vi "bigcryo_H-full_ver2p1.vi"() -> ()   [LabVIEW 2019]
uses:
  Components/B_Globals.vi
  <vilib>/Analysis/NI_AALPro.lvlib
panel:
  in  "Heater On":bool
  in  "Pause Off":bool
  out "Set Field [T]":dbl=0.05
  out "Set Rate [T]":dbl=0.012520565999999999
  out "Exec Time [ms]":u32=400
  out "Stable":bool
  out "Act. Rate [T/min]":dbl=-0.0
  out "Read Buffer":string="15:13:43 OUTPUT: 0.00000 TESLA AT 0.0 VOLTS\r\n"
  in  "stop":bool
  out "Its":i32=50
  out "Running Sequence":bool
  in  "Set Field":dbl
  in  "Rate":dbl=0.05
  in  "Go To":bool
  out "Field [T]":dbl
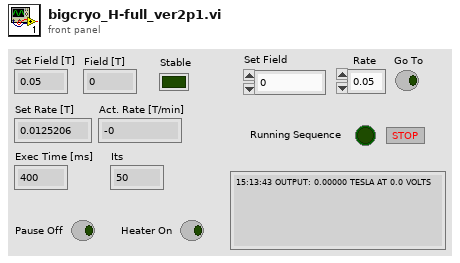
[diagram p1: front panel]
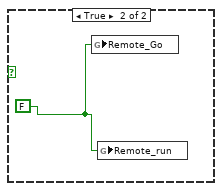
[diagram p2: hidden frame]
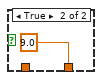
[diagram p5: hidden frame]
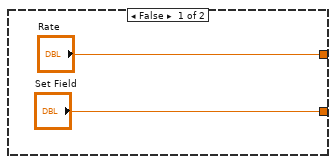
[diagram p7: hidden frame]
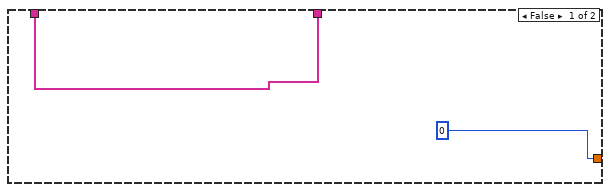
[diagram p9: hidden frame]
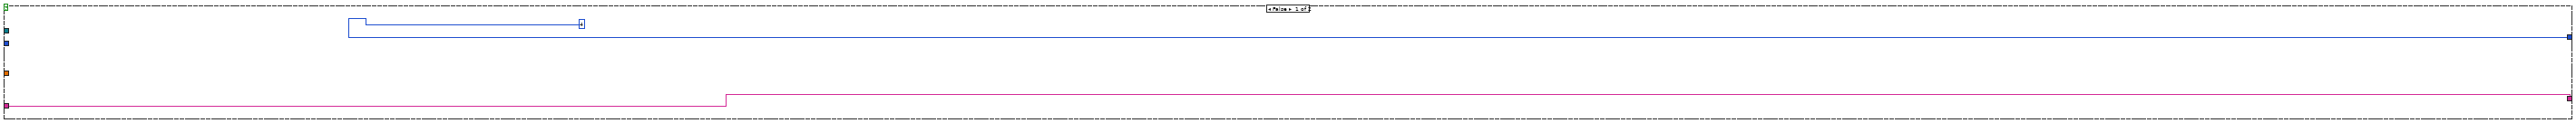
[diagram p12: hidden frame]
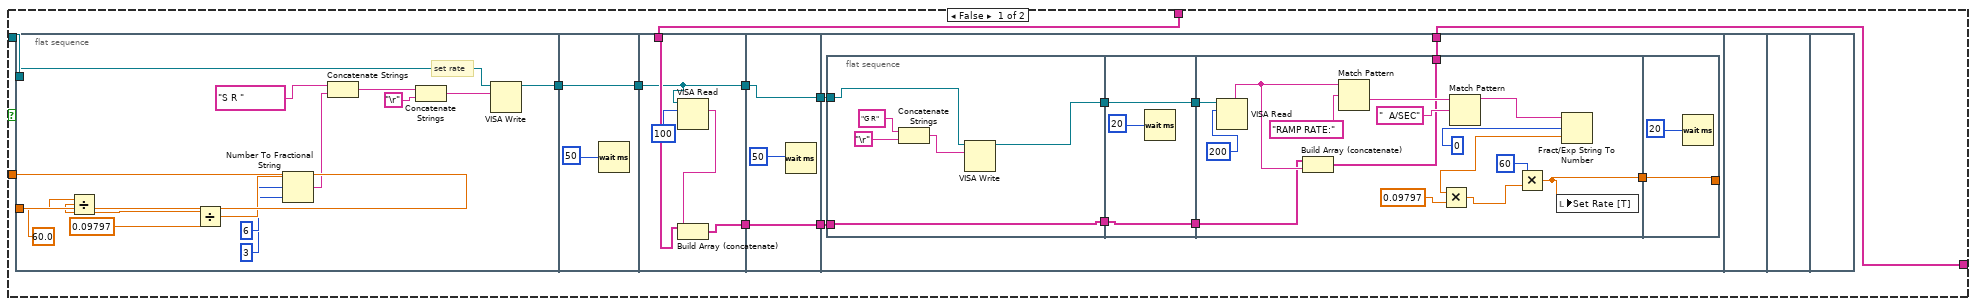
[diagram p13: hidden frame]
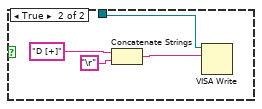
[diagram p17: hidden frame]
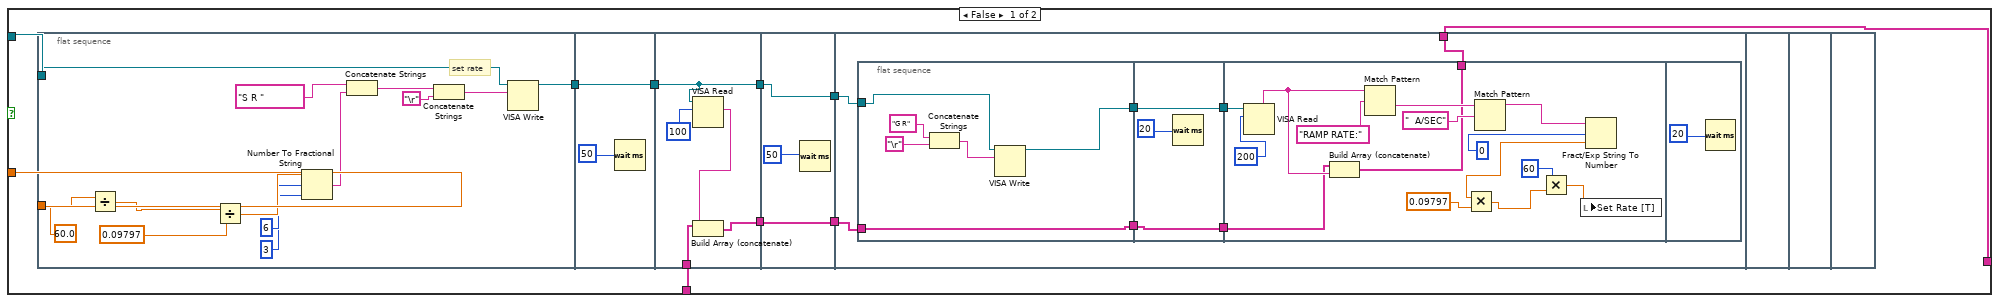
[diagram p18: hidden frame]
diagram:
  n1 = Tick Count (ms)() -> (millisecond timer value=w1:u32)
  n2 = VISA Clear(VISA resource name=refnum<visa-resource-name> "COM6" ("Lakeshore Address")) -> (VISA resource name out=w3:refnum<visa-resource-name>)  [unwired: 1 in, 1 out]
  n3 = while {
    shift-right: [w103] -> _
    shift-left: _ -> [w104]
    shift-right: [w100] -> _
    shift-left: _ -> [w101]
    tunnel: w3 -> [w105]
    shift-right: [w96] -> _
    shift-left: 0 -> [w50]
    shift-right: [w83] -> _
    shift-left: w1 -> [w82]
    shift-right: [w23] -> _
    shift-left: _ -> [w34]
    i -> [w93]
    stop <- FALSE stop-if-true
    n4 = flat-sequence {
      tunnel: w50 -> [w114]
      tunnel: w101 -> [w108]
      tunnel: w104 -> [w110]
      tunnel: w105 -> [w115]
      tunnel: [w115] -> w49
      tunnel: [w111] -> w48
      tunnel: [w107] -> w47
      tunnel: [w114] -> w46
      tunnel: [w106] -> w35
      tunnel: w34 -> [w106]
      tunnel: [w123] -> w87
      tunnel: [w122] -> w86
      tunnel: [w121] -> w85
      tunnel: [w120] -> w84
      tunnel: [w118] -> w83
      tunnel: w82 -> [w117]
      tunnel: w49 -> [w123]
      tunnel: w48 -> [w122]
      tunnel: w47 -> [w121]
      tunnel: w46 -> [w120]
      tunnel: w35 -> [w116]
      tunnel: [w116] -> w31
      tunnel: [w130] -> w45
      tunnel: [w129] -> w43
      tunnel: [w128] -> w41
      tunnel: [w127] -> w39
      tunnel: [w125] -> w37
      tunnel: w87 -> [w130]
      tunnel: w86 -> [w129]
      tunnel: w85 -> [w128]
      tunnel: w84 -> [w127]
      tunnel: [w124] -> w32
      tunnel: w31 -> [w124]
      tunnel: w45 -> [w134]
      tunnel: [w133] -> w44
      tunnel: w43 -> [w138]
      tunnel: [w138] -> w42
      tunnel: w41 -> [w137]
      tunnel: [w137] -> w40
      tunnel: w39 -> [w136]
      tunnel: [w136] -> w38
      tunnel: w37 -> [w135]
      tunnel: [w135] -> w36
      tunnel: [w132] -> w33
      tunnel: w32 -> [w132]
      tunnel: w44 -> [w141]
      tunnel: [w140] -> w92
      tunnel: w42 -> [w148]
      tunnel: [w148] -> w91
      tunnel: w40 -> [w147]
      tunnel: [w147] -> w90
      tunnel: w38 -> [w146]
      tunnel: [w146] -> w89
      tunnel: w36 -> [w145]
      tunnel: [w145] -> w88
      tunnel: w33 -> [w144]
      tunnel: [w144] -> w29
      tunnel: [w198] -> w81
      tunnel: [w197] -> w80
      tunnel: [w195] -> w79
      tunnel: [w196] -> w78
      tunnel: [w191] -> w77
      tunnel: w92 -> [w191]
      tunnel: w91 -> [w198]
      tunnel: w90 -> [w197]
      tunnel: w89 -> [w196]
      tunnel: w88 -> [w195]
      tunnel: [w190] -> w51
      tunnel: [w189] -> w30
      tunnel: w29 -> [w189]
      tunnel: w81 -> [w206]
      tunnel: [w206] -> w76
      tunnel: w80 -> [w205]
      tunnel: [w205] -> w75
      tunnel: w79 -> [w204]
      tunnel: [w204] -> w74
      tunnel: w78 -> [w203]
      tunnel: [w203] -> w73
      tunnel: w77 -> [w202]
      tunnel: [w202] -> w72
      tunnel: [w200] -> w52
      tunnel: w51 -> [w200]
      tunnel: w30 -> [w199]
      tunnel: [w199] -> w27
      tunnel: [w210] -> w71
      tunnel: w76 -> [w221]
      tunnel: [w221] -> w70
      tunnel: w75 -> [w220]
      tunnel: [w220] -> w69
      tunnel: w74 -> [w219]
      tunnel: [w219] -> w68
      tunnel: w73 -> [w218]
      tunnel: [w218] -> w67
      tunnel: w72 -> [w217]
      tunnel: [w217] -> w66
      tunnel: [w209] -> w65
      tunnel: w52 -> [w208]
      tunnel: [w207] -> w28
      tunnel: w27 -> [w207]
      tunnel: [w230] -> w64
      tunnel: [w225] -> w62
      tunnel: [w229] -> w60
      tunnel: [w228] -> w58
      tunnel: [w227] -> w56
      tunnel: [w226] -> w54
      tunnel: w71 -> [w225]
      tunnel: w70 -> [w226]
      tunnel: w69 -> [w228]
      tunnel: w68 -> [w227]
      tunnel: w67 -> [w230]
      tunnel: w66 -> [w229]
      tunnel: w65 -> [w224]
      tunnel: w28 -> [w222]
      tunnel: [w223] -> w25
      tunnel: w64 -> [w238]
      tunnel: [w238] -> w63
      tunnel: w62 -> [w237]
      tunnel: [w237] -> w61
      tunnel: w60 -> [w236]
      tunnel: [w236] -> w59
      tunnel: w58 -> [w235]
      tunnel: [w235] -> w57
      tunnel: w56 -> [w234]
      tunnel: [w234] -> w55
      tunnel: w54 -> [w233]
      tunnel: [w233] -> w53
      tunnel: [w231] -> w26
      tunnel: w25 -> [w231]
      tunnel: [w265] -> w99
      tunnel: [w263] -> w98
      tunnel: [w273] -> w97
      tunnel: w63 -> [w273]
      tunnel: [w268] -> w95
      tunnel: w61 -> [w268]
      tunnel: [w272] -> w94
      tunnel: w59 -> [w272]
      tunnel: w57 -> [w271]
      tunnel: w55 -> [w270]
      tunnel: w53 -> [w269]
      tunnel: w26 -> [w256]
      tunnel: [w256] -> w24
      tunnel: w99 -> [w292]
      tunnel: w98 -> [w291]
      tunnel: w97 -> [w287]
      tunnel: [w292] -> w22
      tunnel: [w291] -> w20
      tunnel: [w286] -> w18
      tunnel: [w285] -> w16
      tunnel: w95 -> [w285]
      tunnel: w94 -> [w284]
      tunnel: [w284] -> w14
      tunnel: [w274] -> w12
      tunnel: [w278] -> w10
      tunnel: [w282] -> w8
      tunnel: w24 -> [w282]
      tunnel: w22 -> [w320]
      tunnel: [w320] -> w21
      tunnel: w20 -> [w319]
      tunnel: [w319] -> w19
      tunnel: w18 -> [w306]
      tunnel: [w306] -> w17
      tunnel: w16 -> [w318]
      tunnel: [w318] -> w15
      tunnel: w14 -> [w315]
      tunnel: [w315] -> w13
      tunnel: w12 -> [w317]
      tunnel: [w317] -> w11
      tunnel: w10 -> [w316]
      tunnel: [w316] -> w9
      tunnel: w8 -> [w314]
      tunnel: [w313] -> w7
      tunnel: [w311] -> w6
      tunnel: [w309] -> w5
      tunnel: [w364] -> w100
      tunnel: [w365] -> w103
      tunnel: w21 -> [w365]
      tunnel: w19 -> [w364]
      tunnel: w17 -> [w358]
      tunnel: [w363] -> w96
      tunnel: w15 -> [w362]
      tunnel: w13 -> [w361]
      tunnel: w11 -> [w360]
      tunnel: w9 -> [w359]
      tunnel: [w357] -> w23
      tunnel: w7 -> [w356]
      tunnel: w6 -> [w355]
      tunnel: w5 -> [w354]
      frame #0 {
        n5 = Array Size(array=w110) -> (size(s)=w113:i32)
        n6 = Subtract(x=w113, y=1000) -> (x-y=w109:i32)
        n7 = Array Subset(array=w110, index=w109) -> (w111:dbl[])  [unwired: 1 in]
        n8 = Array Subset(array=w108, index=w109) -> (w107:dbl[])  [unwired: 1 in]
      }
      frame #1 {
        n9 = Tick Count (ms)() -> (millisecond timer value=w118:u32)
        n10 = Subtract(x=w118, y=w117) -> (x-y=→"Exec Time [ms]":u32)
      }
      frame #2 {
        n11 = case shown="False" "stop" {
          frame False {
          }
          frame True {
            w131 = FALSE
            n12 = global write "B_Globals.vi" "Remote_Go"(w131) -> ()
            n13 = global write "B_Globals.vi" "Remote_run"(w131) -> ()
          }
        }
        n14 = call <vilib>:"High Resolution Relative Seconds.vi"() -> ("relative seconds"=w125:dbl)
      }
      frame #3 {
        n15 = VISA Clear(VISA resource name=w134) -> (VISA resource name out=w133:refnum<visa-resource-name>)  [unwired: 1 in, 1 out]
      }
      frame #4 {
        n16 = case shown="True" "Pause Off" {
          tunnel: w141 -> [w169 w170]
          tunnel: [w169 w173] -> w139
          frame False {
          }
          frame True {
            n17 = flat-sequence {
              tunnel: [w176] -> w172
              tunnel: w170 -> [w175]
              tunnel: w172 -> [w180]
              tunnel: [w180] -> w171
              tunnel: [w185] -> w174
              tunnel: w171 -> [w184]
              tunnel: [w186] -> _
              tunnel: w174 -> [w186]
              tunnel: [w186] -> w173
              frame #0 {
                n18 = Concatenate Strings("P  [0]" ("Command"), "\r") -> (w178:string)
                n19 = VISA Write(VISA resource name=w175, write buffer=w178) -> (VISA resource name out=w176:refnum<visa-resource-name>)  [unwired: 1 in, 2 out]
              }
              frame #1 {
                n20 = Wait (ms)(milliseconds to wait=u32 50 ("Pre Delay")) -> ()  [unwired: 1 out]
              }
              frame #2 {
                n21 = VISA Read(VISA resource name=w184, byte count=u32 200) -> (VISA resource name out=w185:refnum<visa-resource-name>, read buffer=w182:string)  [unwired: 1 in, 2 out]
                n22 = local write "Read Buffer"(w182) -> ()
              }
              frame #3 {
                n23 = Wait (ms)(milliseconds to wait=u32 50 ("Pre Delay")) -> ()  [unwired: 1 out]
                n24 = local write "Pause Off"(FALSE) -> ()
              }
            }
          }
        }
        n25 = case shown="True" "Heater On" {
          tunnel: [w149 w150] -> w140
          tunnel: w139 -> [w149 w151]
          frame False {
          }
          frame True {
            n26 = flat-sequence {
              tunnel: [w156] -> w154
              tunnel: w151 -> [w155]
              tunnel: w154 -> [w160]
              tunnel: [w160] -> w153
              tunnel: [w165] -> w152
              tunnel: w153 -> [w164]
              tunnel: [w166] -> w150
              tunnel: w152 -> [w166]
              tunnel: [w166] -> _
              frame #0 {
                n27 = Concatenate Strings("H  [1]" ("Command"), "\r") -> (w158:string)
                n28 = VISA Write(VISA resource name=w155, write buffer=w158) -> (VISA resource name out=w156:refnum<visa-resource-name>)  [unwired: 1 in, 2 out]
              }
              frame #1 {
                n29 = Wait (ms)(milliseconds to wait=u32 50 ("Pre Delay")) -> ()  [unwired: 1 out]
              }
              frame #2 {
                n30 = VISA Read(VISA resource name=w164, byte count=u32 200) -> (VISA resource name out=w165:refnum<visa-resource-name>, read buffer=w162:string)  [unwired: 1 in, 2 out]
                n31 = local write "Read Buffer"(w162) -> ()
              }
              frame #3 {
                n32 = Wait (ms)(milliseconds to wait=u32 50 ("Pre Delay")) -> ()  [unwired: 1 out]
                n33 = local write "Heater On"(FALSE) -> ()
              }
            }
          }
        }
      }
      frame #5 {
        n34 = Concatenate Strings("G O" ("Command"), "\r") -> (w193:string)
        n35 = VISA Write(VISA resource name=w191, write buffer=w193) -> (VISA resource name out=w190:refnum<visa-resource-name>)  [unwired: 1 in, 2 out]
      }
      frame #6 {
        n36 = Wait (ms)(milliseconds to wait=u32 50 ("Pre Delay")) -> ()  [unwired: 1 out]
      }
      frame #7 {
        n37 = VISA Read(VISA resource name=w208, byte count=u32 200) -> (read buffer=w209:string)  [unwired: 1 in, 3 out]
        n38 = Match Pattern(string=w209, regular expression="OUTPUT:") -> (after substring=w212:string)  [unwired: 1 in, 3 out]
        n39 = Match Pattern(string=w212, regular expression=" TESLA") -> (before substring=w211:string)  [unwired: 1 in, 3 out]
        n40 = Fract/Exp String To Number(string=w211, offset=0) -> (number=w210:dbl)  [unwired: 2 in, 1 out]
      }
      frame #8 {
        n41 = global write "B_Globals.vi" "B [T]"(w225) -> ()
        n42 = Build Array (concatenate)(w222, w224) -> (w223:string[])
        "Field [T]" <- w225
        "Read Buffer" <- w224
      }
      frame #9 {
        n43 = Wait (ms)(milliseconds to wait=u32 50 ("Pre Delay")) -> ()  [unwired: 1 out]
      }
      frame #10 {
        n44 = Build Array (concatenate)(w269, w268) -> (w265:dbl[])
        n45 = Build Array (concatenate)(w271, w270) -> (w263:dbl[])
        n46 = Array Size(array=w265) -> (size(s)=w266:i32)
        n47 = Subtract(x=w266, y=50) -> (x-y=w264:i32)
        n48 = Array Subset(array=w263, index=w264) -> (w261:dbl[])  [unwired: 1 in]
        n49 = Array Subset(array=w265, index=w264) -> (w262:dbl[])  [unwired: 1 in]
        n50 = local read "Set Field [T]"() -> (w250:dbl)
        n51 = call <vilib>:"Linear Fit.vi"("Y"=w262, "X"=w261) -> ("slope"=w258:dbl)  [unwired: 9 in, 4 out]
        n52 = local read "Field [T]"() -> (w248:dbl)
        n53 = Multiply(x=w258, y=60) -> (x*y=w257:dbl)
        "Act. Rate [T/min]" <- w257
        n54 = Absolute Value(x=w250) -> (abs(x)=w249:dbl)
        n55 = Absolute Value(x=w248) -> (abs(x)=w240:dbl)
        n56 = Add(x=1, y=w240) -> (x+y=w239:dbl)
        n57 = Multiply(x=0.008, y=w239) -> (x*y=w246:dbl)
        n58 = Subtract(x=w249, y=w240) -> (x-y=w255:dbl)
        n59 = Absolute Value(x=w257) -> (abs(x)=w259:dbl)
        n60 = Less?(x=w259, y=w246) -> (x < y?=w252:bool)
        n61 = Add(x=1, y=w240) -> (x+y=w242:dbl)
        n62 = Absolute Value(x=w255) -> (abs(x)=w254:dbl)
        n63 = Multiply(x=w242, y=0.008) -> (x*y=w244:dbl)
        n64 = Less?(x=w254, y=w244) -> (x < y?=w251:bool)
        n65 = And(x=w252, y=w251) -> (x .and. y?=w253:bool)
        "Stable" <- w253
        n66 = global write "B_Globals.vi" "Rem_stable_B"(w253) -> ()
      }
      frame #11 {
        n67 = global read "B_Globals.vi" "Remote_Go"() -> (w290:bool)
        n68 = global read "B_Globals.vi" "Remote_run"() -> (w283:bool)
        "Running Sequence" <- w283
        n69 = Or(x=w290, y="Go To") -> (x .or. y?=w288:bool)
        n70 = case shown="True" w288 {
          tunnel: w287 -> [w301 w303]
          tunnel: [w301 w302] -> w286
          frame False {
          }
          frame True {
            n71 = flat-sequence {
              tunnel: w303 -> [_]
              tunnel: [1] -> w302
              frame #0 {
              }
              frame #1 {
                w305 = FALSE
                n72 = local write "Go To"(w305) -> ()
                n73 = global write "B_Globals.vi" "Remote_Go"(w305) -> ()
              }
            }
          }
        }
        n74 = case shown="True" w283 {
          tunnel: ["Set Field" w299] -> w275
          tunnel: ["Rate" w300] -> w279
          frame False {
          }
          frame True {
            n75 = global read "B_Globals.vi" "Remote_Rate"() -> (w300:dbl)
            n76 = global read "B_Globals.vi" "Remote_set"() -> (w299:dbl)
            n77 = local write "Rate"(w300) -> ()
            n78 = local write "Set Field"(w299) -> ()
          }
        }
        n79 = Greater?(x=w279, y=0.5) -> (0:w280:bool)
        n80 = Greater?(x=w275, y=9.0) -> (0:w276:bool)
        n81 = case shown="False" w276 {
          tunnel: [w293 9.0] -> w274
          tunnel: w275 -> [w293 _]
          frame False {
          }
          frame True {
          }
        }
        n82 = case shown="True" w280 {
          tunnel: [w295 0.5] -> w278
          tunnel: w279 -> [w295 _]
          frame False {
          }
          frame True {
          }
        }
      }
      frame #12 {
        n83 = Not Equal?(x=0, y=w306) -> (x != y?=w309:bool)
        n84 = Not Equal?(x=w306, y=2) -> (x != y?=w310:bool)
        n85 = And(x=w309, y=w310) -> (x .and. y?=w308:bool)
        n86 = case shown="True" w308 {
          tunnel: w315 -> [_ w327]
          tunnel: w314 -> [w322 w326]
          tunnel: [w322 w325] -> w313
          tunnel: [0 w323] -> w311
          frame False {
          }
          frame True {
            n87 = flat-sequence {
              tunnel: w327 -> [w331]
              tunnel: [w330] -> w329
              tunnel: w329 -> [w335]
              tunnel: [w335] -> w328
              tunnel: w328 -> [w348]
              tunnel: w326 -> [w345]
              tunnel: [w344] -> w325
              tunnel: [w337] -> w324
              tunnel: [w352] -> w323
              tunnel: w324 -> [w352]
              frame #0 {
                n88 = Concatenate Strings("G R" ("Command"), "\r") -> (w333:string)
                n89 = VISA Write(VISA resource name=w331, write buffer=w333) -> (VISA resource name out=w330:refnum<visa-resource-name>)  [unwired: 1 in, 2 out]
              }
              frame #1 {
                n90 = Wait (ms)(milliseconds to wait=20) -> ()  [unwired: 1 out]
              }
              frame #2 {
                n91 = VISA Read(VISA resource name=w348, byte count=u32 200) -> (read buffer=w346:string)  [unwired: 1 in, 3 out]
                n92 = Build Array (concatenate)(w345, w346) -> (w344:string[])
                n93 = Match Pattern(string=w346, regular expression="RAMP RATE:") -> (after substring=w349:string)  [unwired: 1 in, 3 out]
                n94 = Match Pattern(string=w349, regular expression="  A/SEC") -> (before substring=w342:string)  [unwired: 1 in, 3 out]
                n95 = Fract/Exp String To Number(string=w342, offset=0) -> (number=w340:dbl)  [unwired: 2 in, 1 out]
                n96 = Multiply(x=w340, y=0.09797) -> (x*y=w338:dbl)
                n97 = Multiply(x=60, y=w338) -> (x*y=w337:dbl)
                "Set Rate [T]" <- w337
              }
              frame #3 {
                n98 = Wait (ms)(milliseconds to wait=20) -> ()  [unwired: 1 out]
              }
            }
          }
        }
      }
      frame #13 {
        # "Bnow"
        # "Barray"
        n99 = case shown="4" w358 {
          tunnel: w362 -> [_ w384 w591 _ _]
          tunnel: w358 -> [w368 w377 w588 _ _]
          tunnel: [w368 w376 w587 4 w646] -> w363
          tunnel: w359 -> [_ w369 _ _ w648]
          tunnel: w361 -> [_ w373 _ w600 w644]
          tunnel: w360 -> [_ w374 _ _ w645]
          tunnel: w356 -> [w366 w372 w586 w598 w629]
          tunnel: [w366 w371 w586 w598 w623] -> w357
          tunnel: w355 -> [_ w370 _ _ _]
          tunnel: w354 -> [_ _ _ _ _]
          frame 0, Default {
            n100 = Wait (ms)(milliseconds to wait=0) -> ()  [unwired: 1 out]
          }
          frame 1 {
            # "If True need to reverse polarity"
            n101 = Less Than 0?(x=w374) -> (x < 0?=w375:bool)
            n102 = Number To Fractional String(number=w384) -> (F-format string=w387:string)  [unwired: 3 in]
            n103 = String Subset(string=w387, length (rest)=1 ("length (rest)")) -> (substring=w386:string)  [unwired: 1 in]
            n104 = Equal?(x=w386, y="-") -> (x = y?=w379:bool)
            n105 = Not Or(1:w375, 2:w379) -> (0:w383:bool)
            n106 = Not Or(1:w383, 2:w379) -> (0:w382:bool)
            n107 = Not Or(1:w375, 2:w383) -> (0:w381:bool)
            n108 = Not Or(1:w381, 2:w382) -> (0:w380:bool)
            n109 = Not(x=w380) -> (.not. x?=w378:bool)
            n110 = case shown="True" w378 {
              tunnel: w377 -> [_ _]
              tunnel: [4 2] -> w376
              tunnel: w369 -> [_ w438]
              tunnel: w373 -> [_ w436]
              tunnel: w372 -> [w389 w427]
              tunnel: [w389 w418] -> w371
              tunnel: w370 -> [_ w399]
              tunnel: w369 -> [_ w397]
              frame False {
              }
              frame True {
                n111 = flat-sequence {
                  tunnel: w436 -> [w442]
                  tunnel: [w442] -> w435
                  tunnel: [w443] -> w428
                  tunnel: w427 -> [w443]
                  tunnel: [w441] -> w400
                  tunnel: w399 -> [w441]
                  tunnel: [w446] -> w406
                  tunnel: w435 -> [w446]
                  tunnel: w428 -> [w445]
                  tunnel: [w445] -> w405
                  tunnel: w400 -> [w444]
                  tunnel: [w444] -> w398
                  tunnel: w406 -> [w454]
                  tunnel: [w454] -> w404
                  tunnel: w405 -> [w453]
                  tunnel: [w453] -> w402
                  tunnel: w398 -> [w452]
                  tunnel: w397 -> [w451]
                  tunnel: [w447] -> w396
                  tunnel: w404 -> [w457]
                  tunnel: [w457] -> w403
                  tunnel: w402 -> [w456]
                  tunnel: [w456] -> w401
                  tunnel: w396 -> [w455]
                  tunnel: [w455] -> w395
                  tunnel: [w462] -> w439
                  tunnel: w403 -> [w461]
                  tunnel: [w460] -> w425
                  tunnel: w401 -> [w460]
                  tunnel: [w459] -> w407
                  tunnel: w395 -> [w458]
                  tunnel: [w458] -> w394
                  tunnel: [w473] -> w434
                  tunnel: w439 -> [w473]
                  tunnel: [w472] -> w426
                  tunnel: w425 -> [w472]
                  tunnel: [w471] -> w408
                  tunnel: w407 -> [w471]
                  tunnel: w394 -> [w470]
                  tunnel: [w470] -> w393
                  tunnel: w434 -> [w485]
                  tunnel: [w485] -> w433
                  tunnel: w426 -> [w484]
                  tunnel: [w483] -> w423
                  tunnel: [w475] -> w409
                  tunnel: w408 -> [_]
                  tunnel: w393 -> [w482]
                  tunnel: [w482] -> w392
                  tunnel: w433 -> [w491]
                  tunnel: [w491] -> w432
                  tunnel: [w489] -> w424
                  tunnel: w423 -> [w489]
                  tunnel: [w488] -> w410
                  tunnel: w409 -> [w488]
                  tunnel: w392 -> [w487]
                  tunnel: [w487] -> w391
                  tunnel: w432 -> [w492]
                  tunnel: w438 -> [w497]
                  tunnel: [w492] -> w437
                  tunnel: w424 -> [w493]
                  tunnel: [w494] -> w421
                  tunnel: [w496] -> w411
                  tunnel: w410 -> [w496]
                  tunnel: w391 -> [w495]
                  tunnel: [w569] -> w431
                  tunnel: w437 -> [w569]
                  tunnel: [w568] -> w422
                  tunnel: w421 -> [w568]
                  tunnel: [w567] -> w412
                  tunnel: w411 -> [w567]
                  tunnel: w431 -> [w572]
                  tunnel: [w572] -> w430
                  tunnel: w422 -> [w570]
                  tunnel: [w570] -> w419
                  tunnel: [w571] -> w413
                  tunnel: w412 -> [w571]
                  tunnel: w430 -> [w575]
                  tunnel: [w575] -> w429
                  tunnel: [w574] -> w420
                  tunnel: w419 -> [w574]
                  tunnel: [w573] -> w414
                  tunnel: w413 -> [w573]
                  tunnel: w429 -> [w578]
                  tunnel: w420 -> [w577]
                  tunnel: [w577] -> w417
                  tunnel: [w576] -> w415
                  tunnel: w414 -> [w576]
                  tunnel: w417 -> [w583]
                  tunnel: [w583] -> w416
                  tunnel: w415 -> [w582]
                  tunnel: [w584] -> w418
                  tunnel: w416 -> [w584]
                  frame #0 {
                  }
                  frame #1 {
                  }
                  frame #2 {
                    n112 = Subtract(x=w452, y=w451) -> (x-y=w450:dbl)
                    n113 = Absolute Value(x=w450) -> (abs(x)=w449:dbl)
                    n114 = Less?(x=w449, y=0.01) -> (x < y?=w447:bool)
                  }
                  frame #3 {
                  }
                  frame #4 {
                    w459 = 0.0
                    # "set set field"
                    n115 = Number To Fractional String(number=w459, width (-)=i16 6, precision (6)=i16 3) -> (F-format string=w466:string)  [unwired: 1 in]
                    n116 = Concatenate Strings("S [%][MID] " ("string"), w466) -> (w463:string)
                    n117 = Concatenate Strings(w463, "\r") -> (w465:string)
                    n118 = VISA Write(VISA resource name=w461, write buffer=w465) -> (VISA resource name out=w462:refnum<visa-resource-name>)  [unwired: 1 in, 2 out]
                  }
                  frame #5 {
                    n119 = Wait (ms)(milliseconds to wait=50) -> ()  [unwired: 1 out]
                  }
                  frame #6 {
                    n120 = VISA Read(VISA resource name=w485, byte count=100) -> (read buffer=w476:string)  [unwired: 1 in, 3 out]
                    n121 = Match Pattern(string=w476, regular expression="SETTING:") -> (after substring=w480:string)  [unwired: 1 in, 3 out]
                    n122 = local write "Read Buffer"(w476) -> ()
                    n123 = Match Pattern(string=w480, regular expression=" TESLA") -> (before substring=w481:string)  [unwired: 1 in, 3 out]
                    n124 = Build Array (concatenate)(w484, w476) -> (w483:string[])
                    n125 = Fract/Exp String To Number(string=w481, offset=0) -> (number=w475:dbl)  [unwired: 2 in, 1 out]
                  }
                  frame #7 {
                    n126 = Wait (ms)(milliseconds to wait=50) -> ()  [unwired: 1 out]
                  }
                  frame #8 {
                    n127 = case shown="True" w495 {
                      tunnel: w492 -> [w507 _]
                      tunnel: w497 -> [w506 _]
                      tunnel: w493 -> [w502 w566]
                      tunnel: [w499 w566] -> w494
                      frame False {
                        n128 = flat-sequence {
                          tunnel: w507 -> [w510]
                          tunnel: w506 -> [w509]
                          tunnel: [w508] -> w505
                          tunnel: w505 -> [w523]
                          tunnel: [w523] -> w504
                          tunnel: w504 -> [w525]
                          tunnel: [w525] -> w503
                          tunnel: w502 -> [w526]
                          tunnel: [w524] -> w500
                          tunnel: w503 -> [w529]
                          tunnel: [w530] -> w501
                          tunnel: w500 -> [w530]
                          tunnel: [w529] -> w498
                          tunnel: w501 -> [w536]
                          tunnel: [w533] -> w499
                          tunnel: w498 -> [w532]
                          frame #0 {
                            # "set rate"
                            n129 = Divide(x=w509, y=60.0) -> (x/y=w515:dbl)
                            n130 = Divide(x=w515, y=0.09797) -> (x/y=w513:dbl)
                            n131 = Number To Fractional String(number=w513, width (-)=i16 6, precision (6)=i16 3) -> (F-format string=w518:string)  [unwired: 1 in]
                            n132 = Concatenate Strings("S R " ("string"), w518) -> (w517:string)
                            n133 = Concatenate Strings(w517, "\r") -> (w521:string)
                            n134 = VISA Write(VISA resource name=w510, write buffer=w521) -> (VISA resource name out=w508:refnum<visa-resource-name>)  [unwired: 1 in, 2 out]
                          }
                          frame #1 {
                            n135 = Wait (ms)(milliseconds to wait=50) -> ()  [unwired: 1 out]
                          }
                          frame #2 {
                            n136 = VISA Read(VISA resource name=w525, byte count=100) -> (read buffer=w527:string)  [unwired: 1 in, 3 out]
                            n137 = Build Array (concatenate)(w526, w527) -> (w524:string[])
                          }
                          frame #3 {
                            n138 = Wait (ms)(milliseconds to wait=50) -> ()  [unwired: 1 out]
                          }
                          frame #4 {
                            n139 = flat-sequence {
                              tunnel: [w542] -> w539
                              tunnel: w536 -> [w541]
                              tunnel: [w541] -> w534
                              tunnel: w532 -> [w540]
                              tunnel: w539 -> [w547]
                              tunnel: [w547] -> w538
                              tunnel: [w546] -> w535
                              tunnel: w534 -> [w546]
                              tunnel: w538 -> [w560]
                              tunnel: [w557] -> w533
                              tunnel: [w550] -> w537
                              tunnel: w535 -> [w549]
                              tunnel: [w564] -> _
                              tunnel: w537 -> [w564]
                              frame #0 {
                                n140 = Concatenate Strings("G R" ("Command"), "\r") -> (w544:string)
                                n141 = VISA Write(VISA resource name=w540, write buffer=w544) -> (VISA resource name out=w542:refnum<visa-resource-name>)  [unwired: 1 in, 2 out]
                              }
                              frame #1 {
                                n142 = Wait (ms)(milliseconds to wait=20) -> ()  [unwired: 1 out]
                              }
                              frame #2 {
                                n143 = VISA Read(VISA resource name=w560, byte count=u32 200) -> (read buffer=w558:string)  [unwired: 1 in, 3 out]
                                n144 = Build Array (concatenate)(w549, w558) -> (w557:string[])
                                n145 = Match Pattern(string=w558, regular expression="RAMP RATE:") -> (after substring=w561:string)  [unwired: 1 in, 3 out]
                                n146 = Match Pattern(string=w561, regular expression="  A/SEC") -> (before substring=w555:string)  [unwired: 1 in, 3 out]
                                n147 = Fract/Exp String To Number(string=w555, offset=0) -> (number=w553:dbl)  [unwired: 2 in, 1 out]
                                n148 = Multiply(x=w553, y=0.09797) -> (x*y=w551:dbl)
                                n149 = Multiply(x=60, y=w551) -> (x*y=w550:dbl)
                                n150 = local write "Set Rate [T]"(w550) -> ()
                              }
                              frame #3 {
                                n151 = Wait (ms)(milliseconds to wait=20) -> ()  [unwired: 1 out]
                              }
                            }
                          }
                          frame #5 {
                          }
                          frame #6 {
                          }
                          frame #7 {
                          }
                        }
                      }
                      frame True {
                      }
                    }
                  }
                  frame #9 {
                  }
                  frame #10 {
                  }
                  frame #11 {
                  }
                  frame #12 {
                    # "Go to set field"
                    n152 = Concatenate Strings("R [%][MID]" ("data"), "\r") -> (w581:string)
                    n153 = VISA Write(VISA resource name=w578, write buffer=w581) -> ()  [unwired: 1 in, 3 out]
                  }
                  frame #13 {
                    n154 = global write "B_Globals.vi" "G_B_set[T]"(w582) -> ()
                    "Set Field [T]" <- w582
                  }
                  frame #14 {
                    n155 = Wait (ms)(milliseconds to wait=50) -> ()  [unwired: 1 out]
                  }
                }
              }
            }
          }
          frame 2 {
            # "Awaiting 0 Field"
            n156 = Subtract(x=w591, y=0) -> (x-y=w593:dbl)
            n157 = Absolute Value(x=w593) -> (abs(x)=w590:dbl)
            n158 = Less?(x=w590, y=0.001) -> (x < y?=w589:bool)
            n159 = case shown="True" w589 {
              tunnel: w588 -> [w595 _]
              tunnel: [w595 3] -> w587
              frame False {
              }
              frame True {
                # "Close to 0"
                n160 = Wait (ms)(milliseconds to wait=1000) -> ()  [unwired: 1 out]
              }
            }
          }
          frame 3 {
            n161 = flat-sequence {
              tunnel: w600 -> [w603]
              frame #0 {
                n162 = Wait (ms)(milliseconds to wait=500) -> ()  [unwired: 1 out]
              }
              frame #1 {
                # "Switch polarity"
                n163 = case shown="False" TRUE {
                  tunnel: w603 -> [_ w604]
                  frame False {
                  }
                  frame True {
                    n164 = Concatenate Strings("D [+]" ("data"), "\r") -> (w607:string)
                    n165 = VISA Write(VISA resource name=w604, write buffer=w607) -> ()  [unwired: 1 in, 3 out]
                  }
                }
              }
              frame #2 {
              }
              frame #3 {
              }
              frame #4 {
                n166 = Wait (ms)(milliseconds to wait=500) -> ()  [unwired: 1 out]
              }
            }
          }
          frame 4 {
            n167 = flat-sequence {
              tunnel: w644 -> [w651]
              tunnel: [w651] -> w642
              tunnel: [w650] -> w631
              tunnel: w629 -> [w650]
              tunnel: [w653] -> w643
              tunnel: w642 -> [w653]
              tunnel: w631 -> [w652]
              tunnel: [w652] -> w630
              tunnel: [w657] -> w649
              tunnel: w645 -> [w655]
              tunnel: w643 -> [w658]
              tunnel: [w656] -> w633
              tunnel: w630 -> [w656]
              tunnel: [w655] -> w617
              tunnel: [w668] -> w641
              tunnel: w649 -> [w668]
              tunnel: w633 -> [w667]
              tunnel: [w667] -> w632
              tunnel: [w666] -> w618
              tunnel: w617 -> [w666]
              tunnel: w641 -> [w680]
              tunnel: [w680] -> w640
              tunnel: [w678] -> w635
              tunnel: w632 -> [w677]
              tunnel: w618 -> [_]
              tunnel: [w670] -> w609
              tunnel: [w685] -> w613
              tunnel: [w684] -> w612
              tunnel: [w683] -> w611
              tunnel: [w682] -> w610
              tunnel: w648 -> [w682]
              tunnel: w635 -> [w684]
              tunnel: w640 -> [w685]
              tunnel: w609 -> [w683]
              tunnel: w613 -> [w694]
              tunnel: [w694] -> w616
              tunnel: w612 -> [w693]
              tunnel: [w692] -> w615
              tunnel: w611 -> [w695]
              tunnel: [w695] -> w614
              tunnel: w610 -> [w687]
              tunnel: w616 -> [w765]
              tunnel: [w765] -> w637
              tunnel: [w764] -> w634
              tunnel: w615 -> [w764]
              tunnel: [w763] -> w619
              tunnel: w614 -> [w763]
              tunnel: w637 -> [w768]
              tunnel: [w768] -> w636
              tunnel: w634 -> [w767]
              tunnel: [w767] -> w624
              tunnel: [w766] -> w620
              tunnel: w619 -> [w766]
              tunnel: [w771] -> w647
              tunnel: w636 -> [w771]
              tunnel: [w770] -> w625
              tunnel: w624 -> [w770]
              tunnel: [w769] -> w621
              tunnel: w620 -> [w769]
              tunnel: w647 -> [w776]
              tunnel: [0] -> w646
              tunnel: [w774] -> w638
              tunnel: [w773] -> w626
              tunnel: w625 -> [w773]
              tunnel: [w772] -> w622
              tunnel: w621 -> [w772]
              tunnel: [w782] -> w639
              tunnel: w638 -> [w782]
              tunnel: [w781] -> w627
              tunnel: w626 -> [w781]
              tunnel: w622 -> [w780]
              tunnel: w639 -> [_]
              tunnel: [w784] -> w628
              tunnel: w627 -> [w784]
              tunnel: [w785] -> w623
              tunnel: w628 -> [w785]
              frame #0 {
              }
              frame #1 {
                n168 = Wait (ms)(milliseconds to wait=50) -> ()  [unwired: 1 out]
              }
              frame #2 {
                # "set set field"
                n169 = Number To Fractional String(number=w655, width (-)=i16 6, precision (6)=i16 3) -> (F-format string=w662:string)  [unwired: 1 in]
                n170 = Concatenate Strings("S [%][MID] " ("string"), w662) -> (w659:string)
                n171 = Concatenate Strings(w659, "\r") -> (w661:string)
                n172 = VISA Write(VISA resource name=w658, write buffer=w661) -> (VISA resource name out=w657:refnum<visa-resource-name>)  [unwired: 1 in, 2 out]
              }
              frame #3 {
                n173 = Wait (ms)(milliseconds to wait=50) -> ()  [unwired: 1 out]
              }
              frame #4 {
                n174 = VISA Read(VISA resource name=w680, byte count=100) -> (read buffer=w671:string)  [unwired: 1 in, 3 out]
                n175 = Build Array (concatenate)(w677, w671) -> (w678:string[])
                n176 = local write "Read Buffer"(w671) -> ()
                n177 = Match Pattern(string=w671, regular expression="SETTING:") -> (after substring=w675:string)  [unwired: 1 in, 3 out]
                n178 = Match Pattern(string=w675, regular expression=" TESLA") -> (before substring=w676:string)  [unwired: 1 in, 3 out]
                n179 = Fract/Exp String To Number(string=w676, offset=0) -> (number=w670:dbl)  [unwired: 2 in, 1 out]
              }
              frame #5 {
                n180 = Wait (ms)(milliseconds to wait=50) -> ()  [unwired: 1 out]
              }
              frame #6 {
                n181 = local read "Set Rate [T]"() -> (w688:dbl)
                n182 = Subtract(x=w688, y=w687) -> (x-y=w691:dbl)
                n183 = Absolute Value(x=w691) -> (abs(x)=w690:dbl)
                n184 = Less?(x=w690, y=0.01) -> (x < y?=w686:bool)
                n185 = case shown="True" w686 {
                  tunnel: w694 -> [w705 _]
                  tunnel: w687 -> [w704 _]
                  tunnel: [w698 w762] -> w692
                  tunnel: w693 -> [w696 w762]
                  frame False {
                    n186 = flat-sequence {
                      tunnel: w705 -> [w708]
                      tunnel: w704 -> [w707]
                      tunnel: [w706] -> w703
                      tunnel: w703 -> [w721]
                      tunnel: [w721] -> w702
                      tunnel: w702 -> [w724]
                      tunnel: [w724] -> w701
                      tunnel: [w723] -> w699
                      tunnel: w696 -> [w722]
                      tunnel: w701 -> [w727]
                      tunnel: [w728] -> w700
                      tunnel: w699 -> [w728]
                      tunnel: [w727] -> w697
                      tunnel: w700 -> [w734]
                      tunnel: [w731] -> w698
                      tunnel: w697 -> [w730]
                      frame #0 {
                        # "set rate"
                        n187 = Divide(x=w707, y=60.0) -> (x/y=w713:dbl)
                        n188 = Divide(x=w713, y=0.09797) -> (x/y=w711:dbl)
                        n189 = Number To Fractional String(number=w711, width (-)=i16 6, precision (6)=i16 3) -> (F-format string=w716:string)  [unwired: 1 in]
                        n190 = Concatenate Strings("S R " ("string"), w716) -> (w715:string)
                        n191 = Concatenate Strings(w715, "\r") -> (w719:string)
                        n192 = VISA Write(VISA resource name=w708, write buffer=w719) -> (VISA resource name out=w706:refnum<visa-resource-name>)  [unwired: 1 in, 2 out]
                      }
                      frame #1 {
                        n193 = Wait (ms)(milliseconds to wait=50) -> ()  [unwired: 1 out]
                      }
                      frame #2 {
                        n194 = VISA Read(VISA resource name=w724, byte count=100) -> (read buffer=w725:string)  [unwired: 1 in, 3 out]
                        n195 = Build Array (concatenate)(w722, w725) -> (w723:string[])
                      }
                      frame #3 {
                        n196 = Wait (ms)(milliseconds to wait=50) -> ()  [unwired: 1 out]
                      }
                      frame #4 {
                        n197 = flat-sequence {
                          tunnel: [w739] -> w736
                          tunnel: w734 -> [w738]
                          tunnel: [w738] -> w732
                          tunnel: w730 -> [w737]
                          tunnel: w736 -> [w744]
                          tunnel: [w744] -> w735
                          tunnel: [w743] -> w733
                          tunnel: w732 -> [w743]
                          tunnel: w735 -> [w757]
                          tunnel: [w754] -> w731
                          tunnel: w733 -> [w747]
                          frame #0 {
                            n198 = Concatenate Strings("G R" ("Command"), "\r") -> (w741:string)
                            n199 = VISA Write(VISA resource name=w737, write buffer=w741) -> (VISA resource name out=w739:refnum<visa-resource-name>)  [unwired: 1 in, 2 out]
                          }
                          frame #1 {
                            n200 = Wait (ms)(milliseconds to wait=20) -> ()  [unwired: 1 out]
                          }
                          frame #2 {
                            n201 = VISA Read(VISA resource name=w757, byte count=u32 200) -> (read buffer=w755:string)  [unwired: 1 in, 3 out]
                            n202 = Build Array (concatenate)(w747, w755) -> (w754:string[])
                            n203 = Match Pattern(string=w755, regular expression="RAMP RATE:") -> (after substring=w758:string)  [unwired: 1 in, 3 out]
                            n204 = Match Pattern(string=w758, regular expression="  A/SEC") -> (before substring=w752:string)  [unwired: 1 in, 3 out]
                            n205 = Fract/Exp String To Number(string=w752, offset=0) -> (number=w750:dbl)  [unwired: 2 in, 1 out]
                            n206 = Multiply(x=w750, y=0.09797) -> (x*y=w748:dbl)
                            n207 = Multiply(x=60, y=w748) -> (x*y=w746:dbl)
                            n208 = local write "Set Rate [T]"(w746) -> ()
                          }
                          frame #3 {
                            n209 = Wait (ms)(milliseconds to wait=20) -> ()  [unwired: 1 out]
                          }
                        }
                      }
                      frame #5 {
                      }
                      frame #6 {
                      }
                      frame #7 {
                      }
                    }
                  }
                  frame True {
                  }
                }
              }
              frame #7 {
              }
              frame #8 {
              }
              frame #9 {
              }
              frame #10 {
                # "Go to set field"
                n210 = Concatenate Strings("R [%][MID]" ("data"), "\r") -> (w779:string)
                n211 = VISA Write(VISA resource name=w776, write buffer=w779) -> (VISA resource name out=w774:refnum<visa-resource-name>)  [unwired: 1 in, 2 out]
              }
              frame #11 {
                n212 = local write "Set Field [T]"(w780) -> ()
                n213 = global write "B_Globals.vi" "G_B_set[T]"(w780) -> ()
              }
              frame #12 {
                n214 = Wait (ms)(milliseconds to wait=50) -> ()  [unwired: 1 out]
              }
              frame #13 {
              }
            }
          }
        }
      }
    }
    "Its" <- w93
  }
